vi "gen_i0X_data.vi"(0 "Processed Image Data In":T4, 2 "Raw Image Data In":T3, 7 "Input data":T1, 11 "Error In":errorcluster) -> (4 "Processed Image Data Out":T4, 12 "A Counts":u32, 14 "B Counts":u32, 15 "Error Out":errorcluster)   [LabVIEW 2023]
uses:
  <vilib>/vision/Image Controls.llb/IMAQ Image.ctl
panel:
  out "Raw Image Data Out":T3
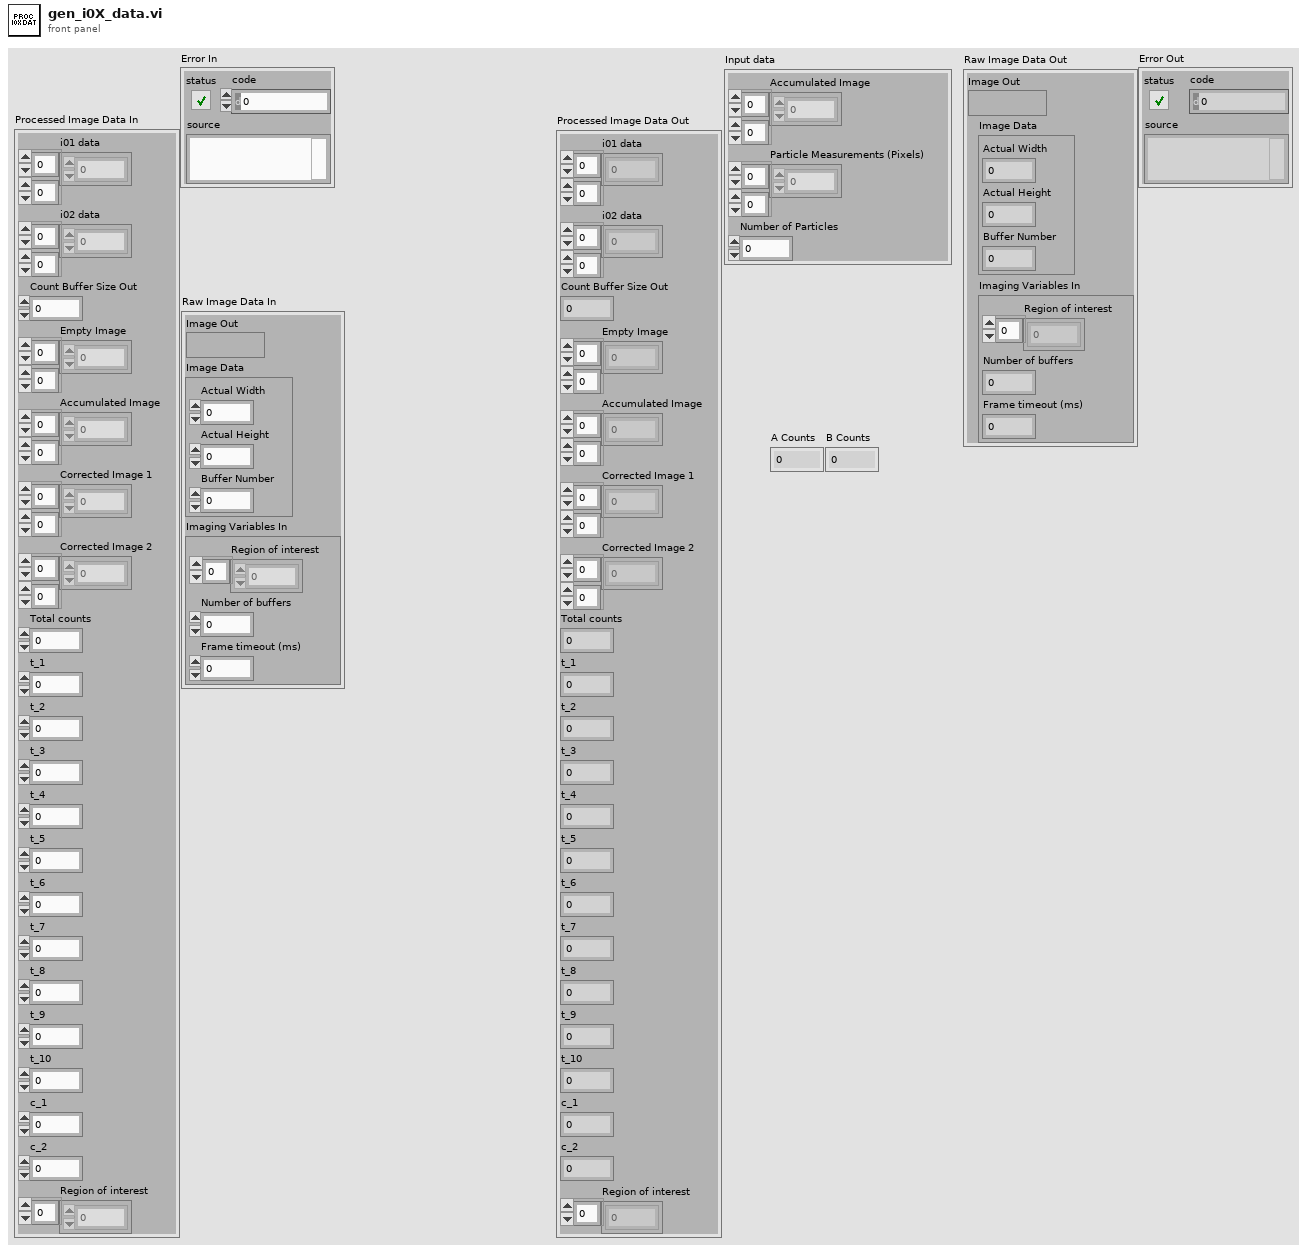
[diagram p1: front panel]
types:
  T1 = cluster{"Accumulated Image":i16[][], "Particle Measurements (Pixels)":dbl[][], "Number of Particles":u16}
  T2 = typedef "IMAQ Image.ctl" = refnum<image>
  T3 = cluster{"Image Out":T2, "Image Data":cluster{"Actual Width":u32, "Actual Height":u32, "Buffer Number":i32}, "Imaging Variables In":cluster{"Region of interest":i32[], "Number of buffers":u32, "Frame timeout (ms)":u32}}
  T4 = cluster{"i01 data":sgl[][], "i02 data":sgl[][], "Count Buffer Size Out":i32, "Empty Image":i16[][], "Accumulated Image":i16[][], "Corrected Image 1":i16[][], "Corrected Image 2":i16[][], "Total counts":i32, "t_1":i32, "t_2":i32, "t_3":i32, "t_4":i32, "t_5":i32, "t_6":i32, "t_7":i32, "t_8":i32, "t_9":i32, "t_10":i32, "c_1":i32, "c_2":i32, "Region of interest":i32[]}
  T5 = cluster{"Actual Width":u32, "Actual Height":u32, "Buffer Number":i32}
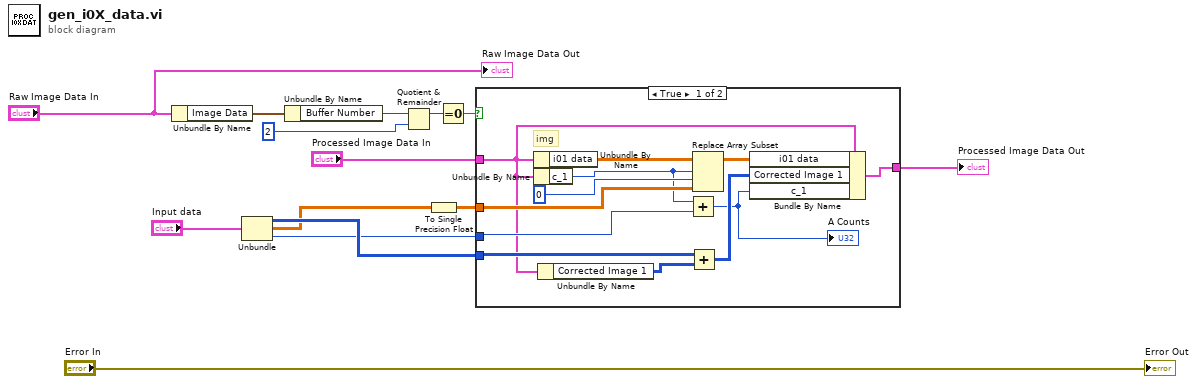
[diagram p0: block diagram]
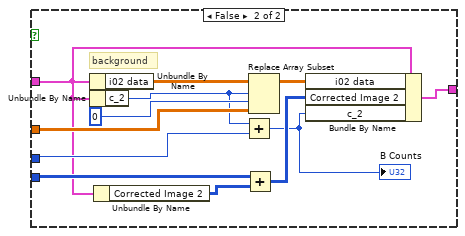
[diagram p2: hidden frame]
diagram:
  n1 = Unbundle By Name("Raw Image Data In") -> ("Image Data"=w7:T5)
  n2 = Unbundle("Input data") -> ("Accumulated Image"=w5:i16[][], "Particle Measurements (Pixels)"=w4:dbl[][], "Number of Particles"=w3:u16)
  n3 = Unbundle By Name(w7) -> ("Buffer Number"=w13:i32)
  n4 = Quotient & Remainder(x=w13, y=2) -> (x-y*floor(x/y)=w12:i32)  [unwired: 1 out]
  n5 = To Single Precision Float(number=w4) -> (single precision float=w11:sgl[][])
  n6 = Equal To 0?(x=w12) -> (x = 0?=w14:bool)
  n7 = case shown="True" w14 {
    tunnel: "Processed Image Data In" -> [w18 w30]
    tunnel: w11 -> [w24 w36]
    tunnel: w3 -> [w21 w33]
    tunnel: w5 -> [w20 w32]
    tunnel: [w16 w28] -> w9
    frame True {
      # "img"
      n8 = Unbundle By Name(w18) -> ("i01 data"=w26:sgl[][])
      n9 = Unbundle By Name(w18) -> ("c_1"=w22:i32)
      n10 = Unbundle By Name(w18) -> ("Corrected Image 1"=w19:i16[][])
      n11 = Add(x=w22, y=w21) -> (x+y=w15:i32)
      "A Counts" <- w15
      n12 = Add(x=w20, y=w19) -> (x+y=w17:i16[][])
      n13 = Replace Array Subset(array=w26, new element=w24, index (row)=w22, index (col)=0 ("disabled index (col)")) -> (w23:sgl[][])
      n14 = Bundle By Name(cluster=w18, "i01 data"=w23, "Corrected Image 1"=w17, "c_1"=w15) -> (w16:T4)
    }
    frame False {
      # "background"
      n15 = Unbundle By Name(w30) -> ("i02 data"=w38:sgl[][])
      n16 = Unbundle By Name(w30) -> ("c_2"=w34:i32)
      n17 = Unbundle By Name(w30) -> ("Corrected Image 2"=w31:i16[][])
      n18 = Add(x=w34, y=w33) -> (x+y=w27:i32)
      "B Counts" <- w27
      n19 = Add(x=w32, y=w31) -> (x+y=w29:i16[][])
      n20 = Replace Array Subset(array=w38, new element=w36, index (row)=w34, index (col)=0 ("disabled index (col)")) -> (w35:sgl[][])
      n21 = Bundle By Name(cluster=w30, "i02 data"=w35, "Corrected Image 2"=w29, "c_2"=w27) -> (w28:T4)
    }
  }
  "Processed Image Data Out" <- w9
  "Raw Image Data Out" <- "Raw Image Data In"
  "Error Out" <- "Error In"
